vi "test_vision.vi"(11 "cam-id":T1="cam2") -> ()   [LabVIEW 2019]
uses:
  <vilib>/userDefined/High Color/IMAQdx.ctl
  Ctrl/clamp-result_cmd.ctl
  <vilib>/vision/driver/NI_Vision_Acquisition_Software.lvlib
  <resource>/objmgr/IMAQImage.rc
  <vilib>/vision/NI_Vision_Development_Module.lvlib
panel:
  in  "camera file":path
  in  "Reset":bool
  out "error out":errorcluster
  out "Steer Direction":dbl(slide)=22.0 scale=-30.0..30.0
  in  "weight_hor":dbl=0.5
  in  "camera_attrib":cluster{"brightness":u16, "exposure":dbl}={"brightness"=46, "exposure"=0.00510204081632653} {"exposure" scale=0.0..0.25; "brightness" scale=0.0..255.0}
  out "frame dt":u32=40
  out "loop n":i32=2970
  out "x-center":dbl=432.0
  out "dir-chart":cluster{dbl, "max angle":dbl}(graph)
  in  "Tab Control":T2(tab)
  out "dir-data":cluster{"Distance":sgl, "weight-dir":dbl}={"Distance"=506.17236, "weight-dir"=21.90533447265625} {"Distance" format="%.1f"; "weight-dir" format="%.1f"}
  in  "vertual speed":dbl(slide) scale=0.0..200.0
  out "Image roi-in":T3(plugin-control)
  out "Edge Coordinates":cluster{"X":sgl, "Y":sgl}[](array[cluster])=[{"X"=222.72447, "Y"=188.0}, {"X"=728.89685, "Y"=188.0}] {"Y" format="%.1f"; "X" format="%.1f"}
  in  "Clamp Settings":T4={"Contrast"=40, "Filter width"=4, "Steepness"=2, "Subsampling Ratio"=13, "Show Search Area"=TRUE, "Show Search Lines"=TRUE, "Show Edges Found"=TRUE, "Show Result"=TRUE}
  out "Image":T3(plugin-control)
  in  "Color Plane 2":i32(ring)=1 items=["Red", "Green", "Blue", "Hue", "Saturation", "Luminance", "Value", "Intensity"]
  out "ROI-clamp":T5={"Global Rectangle"=[62, 188, 838, 318], "Contours"=[{"Contour Type"=0, "ROI Type"=3, "Points"=[62, 188, 838, 318]}]}
  out "Image Size":cluster{"x":i32, "y":i32}={"x"=864, "y"=480}
  in  "stop":bool
  # "Camera ROI setting"
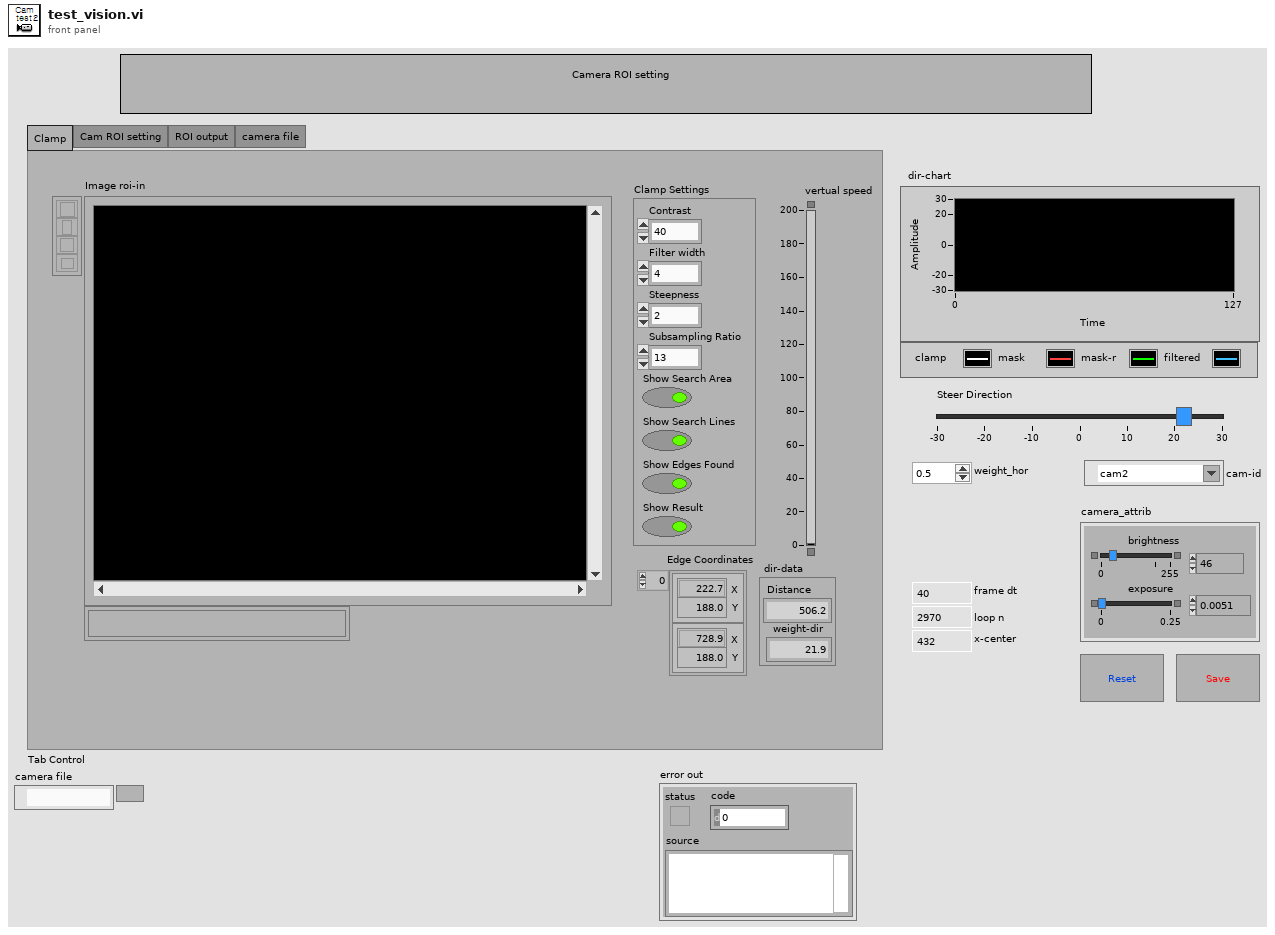
[diagram p1: front panel]
types:
  T1 = typedef "IMAQdx.ctl" = refnum<k21>
  T2 = enum32{"Clamp", "Cam ROI setting", "ROI output", "camera file"}
  T3 = typedef "IMAQ Image.ctl" = refnum<image>
  T4 = cluster{"Contrast":i32, "Filter width":i32, "Steepness":i32, "Subsampling Ratio":u32, "Show Search Area":bool, "Show Search Lines":bool, "Show Edges Found":bool, "Show Result":bool}
  T5 = cluster{"Global Rectangle":i32[], "Contours":cluster{"Contour Type":u32, "ROI Type":u32, "Points":i32[]}[]}
  T6 = typedef "clamp-result_cmd.ctl" = enum16{"write_clamp_overlay-result", "write_center-distance", "write_clamp_result", "write_threshold_result", "read"}
  T7 = typedef "IMAQ Rectangle" = cluster{"Left":i32, "Top":i32, "Right":i32, "Bottom":i32, "Rotation":dbl}
  T8 = typedef "ROI Descriptor" = cluster{"Global Rectangle":i32[], "Contours":cluster{"ID":enum32{"External", "Internal"}, "Type":u32, "Coordinates":i32[]}[]}
  T9 = cluster{"Points":cluster{"X":sgl, "Y":sgl}[], cluster{"X":sgl, "Y":sgl}[], cluster{cluster{"X":sgl, "Y":sgl}, cluster{"X":sgl, "Y":sgl}}[], "Perpendicular Lines":cluster{cluster{"X":sgl, "Y":sgl}, cluster{"X":sgl, "Y":sgl}}[], "ROI Descriptor out":T8}
  T10 = cluster{"Edge Coordinates":cluster{"X":sgl, "Y":sgl}[], "dir-data":cluster{"Distance":sgl, "weight-dir":dbl}, "clamp_result":cluster{"Points":cluster{"X":sgl, "Y":sgl}[], cluster{"X":sgl, "Y":sgl}[], cluster{cluster{"X":sgl, "Y":sgl}, cluster{"X":sgl, "Y":sgl}}[], "Perpendicular Lines":cluster{cluster{"X":sgl, "Y":sgl}, cluster{"X":sgl, "Y":sgl}}[], "ROI Descriptor out":T8}}
  T11 = cluster{"Edge Coordinates":cluster{"X":sgl, "Y":sgl}[], "dir-data":cluster{"Distance":sgl, "weight-dir":dbl}, "clamp_result":cluster{"Points-1":cluster{"X":sgl, "Y":sgl}[], "Points-2":cluster{"X":sgl, "Y":sgl}[], "Points-3":cluster{cluster{"X":sgl, "Y":sgl}, cluster{"X":sgl, "Y":sgl}}[], "Perpendicular Lines":cluster{cluster{"X":sgl, "Y":sgl}, cluster{"X":sgl, "Y":sgl}}[], "ROI Descriptor out":T8}}
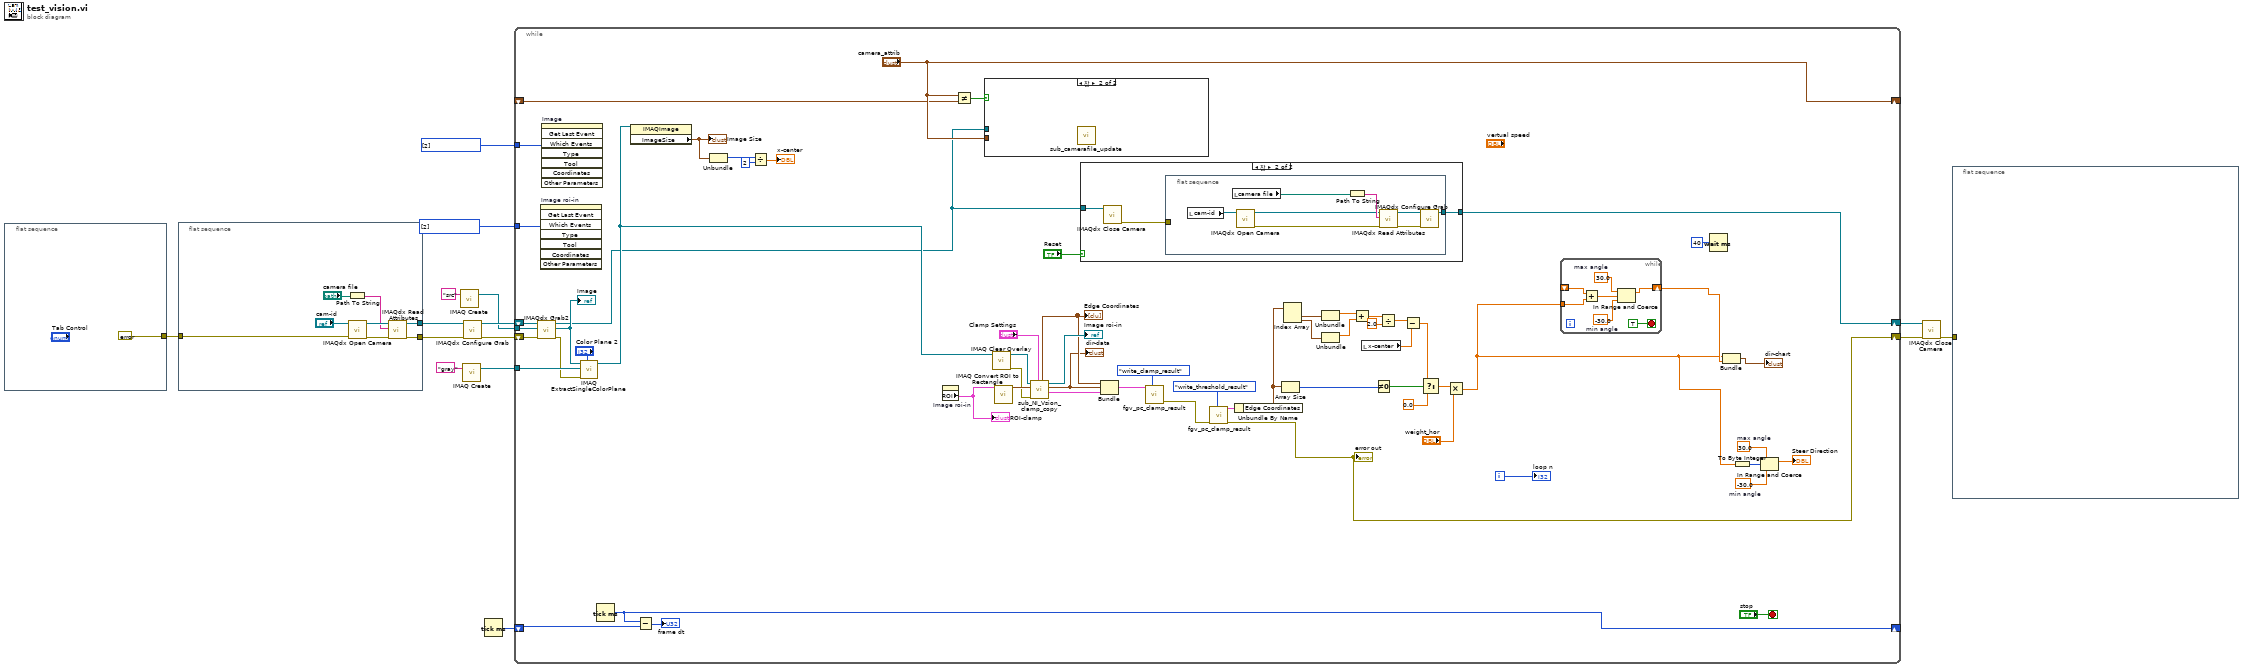
[diagram p0: block diagram]
diagram:
  w9 = i32[] [2] items=["No Event"=0, "Click Event"=1, "Draw Event"=2, "Size Event"=4, "Scroll Event"=5, "Double Click Event"=8] ("Which Events")
  w12 = i32[] [2] items=["No Event"=0, "Click Event"=1, "Draw Event"=2, "Size Event"=4, "Scroll Event"=5, "Double Click Event"=8] ("Which Events")
  n1 = flat-sequence {
    tunnel: [errorcluster {"status"=FALSE, "code"=0, "source"=""} ("error in")] -> w6
    frame #0 {
    }
  }
  n2 = flat-sequence {
    tunnel: [w22] -> w4
    tunnel: [w21] -> w10
    tunnel: w6 -> [w18]
    frame #0 {
      n3 = Path To String(path="camera file") -> (string=w20:string)
      n4 = call <vilib>:"IMAQdx Open Camera.vi"("error in"=w18, "Session In"="cam-id") -> ("error out"=w23:errorcluster, "Session Out"=w24:T1)  [unwired: 8 in]
      n5 = call <vilib>:"IMAQdx Read Attributes.vi"("error in"=w23, "Filename"=w20, "Session In"=w24) -> ("error out"=w21:errorcluster, "Session Out"=w22:T1)  [unwired: 7 in]
    }
  }
  n6 = call "IMAQ Create"("Image Name"="src") -> ("New Image"=w5:T3)  [unwired: 4 in, 1 out]
  n7 = call "IMAQ Create"("Image Name"="gray") -> ("New Image"=w13:T3)  [unwired: 4 in, 1 out]
  n8 = call <vilib>:"IMAQdx Configure Grab.vi"("error in"=w10, "Session In"=w4) -> ("error out"=w3:errorcluster, "Session Out"=w11:T1)  [unwired: 8 in]
  n9 = Tick Count (ms)() -> (millisecond timer value=w8:u32)
  n10 = while {
    tunnel: w5 -> [w83]
    tunnel: w13 -> [w64]
    tunnel: w12 -> [w87]
    tunnel: w9 -> [w81]
    shift-right: [w78] -> _
    shift-left: w8 -> [w79]
    shift-right: ["camera_attrib"] -> _
    shift-left: _ -> [w71]
    shift-right: [w31] -> w2
    shift-left: w11 -> [w82]
    shift-right: [w27] -> w1
    shift-left: w3 -> [w38]
    i -> [w84]
    stop <- "stop" stop-if-true
    w69 = -30.0  # min angle
    w68 = 30.0  # max angle
    n11 = call <vilib>:"IMAQdx Grab2.vi"("error in"=w38, "Image In"=w83, "Session In"=w82) -> ("error out"=w35:errorcluster, "Image Out"=w80:T3, "Session Out"=w32:T1)  [unwired: 5 in, 1 out]
    "Image" <- w80
    n12 = invoke on="Image roi-in" class="ImageControl" method="Get Last Event"("Which Events"=w81) -> ()  [unwired: 7 in, 8 out]
    n13 = invoke on="Image" class="ImageControl" method="Get Last Event"("Which Events"=w87) -> ()  [unwired: 7 in, 8 out]
    n14 = call "IMAQ ExtractSingleColorPlane"("Color Plane"="Color Plane 2", "error in (no error)"=w35, "Image Dst"=w64, "Image Src"=w80) -> ("Image Dst Out"=w36:T3)  [unwired: 6 in, 1 out]
    n15 = Tick Count (ms)() -> (millisecond timer value=w78:u32)
    n16 = property class="IMAQImage"(reference=w36) -> ("ImageSize"=w75:cluster{"x":i32, "y":i32})  [unwired: 1 in, 2 out]
    "Image Size" <- w75
    n17 = Subtract(x=w78, y=w79) -> (x-y=→"frame dt":u32)
    n18 = Unbundle(w75) -> ("x"=w76:i32)  [unwired: 1 out]
    n19 = Divide(x=w76, y=2) -> (x/y=→"x-center":dbl)
    n20 = property on="Image roi-in" class="ImageControl"() -> ("ROI"=w65:T5)  [unwired: 2 in, 2 out]
    "ROI-clamp" <- w65
    n21 = Not Equal?(x="camera_attrib", y=w71) -> (x != y?=w70:bool)
    n22 = case shown="참" w70 {
      tunnel: "camera_attrib" -> [_ _]
      tunnel: w32 -> [_ _]
      frame False {
      }
      frame True {
        n23 = call "sub_camerafile_update.vi"() -> ()  [unwired: 12 in]
      }
    }
    n24 = call "IMAQ Clear Overlay"("Image"=w36) -> ("error out"=w37:errorcluster, "Image Out"=w59:T3)  [unwired: 9 in]
    n25 = call "IMAQ Convert ROI to Rectangle"("ROI Descriptor"=w65) -> ("Rectangle"=w62:T7)  [unwired: 8 in, 1 out]
    n26 = call "sub_NI_Vsion_clamp_copy.vi"("Settings"="Clamp Settings", "error in (no error)"=w37, "Rectangle"=w62, "Image"=w59) -> ("clamp_result"=w58:T9, "dir-data"=w28:cluster{"Distance":sgl, "weight-dir":dbl}, "Image Out"=→"Image roi-in":T3, "Edge Coordinates"=w56:cluster{"X":sgl, "Y":sgl}[])  [unwired: 3 in, 1 out]
    "Edge Coordinates" <- w56
    "dir-data" <- w28
    n27 = case shown="참" "Reset" {
      tunnel: w32 -> [w88 w91]
      tunnel: [w88 w90] -> w31
      frame False {
      }
      frame True {
        n28 = call <vilib>:"IMAQdx Close Camera.vi"("Session In"=w91) -> ("error out"=w89:errorcluster)  [unwired: 10 in]
        n29 = flat-sequence {
          tunnel: [w95] -> w90
          tunnel: w89 -> [_]
          frame #0 {
            n30 = local read "cam-id"() -> (w99:T1)
            n31 = local read "camera file"() -> (w92:path)
            n32 = call <vilib>:"IMAQdx Open Camera.vi"("Session In"=w99) -> ("error out"=w94:errorcluster, "Session Out"=w93:T1)  [unwired: 9 in]
            n33 = Path To String(path=w92) -> (string=w98:string)
            n34 = call <vilib>:"IMAQdx Read Attributes.vi"("error in"=w94, "Filename"=w98, "Session In"=w93) -> ("error out"=w96:errorcluster, "Session Out"=w97:T1)  [unwired: 7 in]
            n35 = call <vilib>:"IMAQdx Configure Grab.vi"("error in"=w96, "Session In"=w97) -> ("Session Out"=w95:T1)  [unwired: 8 in, 1 out]
          }
        }
      }
    }
    n36 = Bundle("Edge Coordinates"=w56, "dir-data"=w28, "clamp_result"=w58) -> (w55:T10)  [unwired: 1 in]
    n37 = call "fgv_pc_clamp_result.vi"("cmd"=clamp-result_cmd."write_clamp_result", "clamp result in"=w55) -> ("error out"=w57:errorcluster)  [unwired: 6 in, 3 out]
    n38 = call "fgv_pc_clamp_result.vi"("cmd"=clamp-result_cmd."write_threshold_result", "error in"=w57) -> ("error out"=w27:errorcluster, "clamp result out"=w54:T11)  [unwired: 6 in, 2 out]
    "error out" <- w27
    n39 = Unbundle By Name(w54) -> ("Edge Coordinates"=w45:cluster{"X":sgl, "Y":sgl}[])
    n40 = Array Size(array=w45) -> (size(s)=w44:i32)
    n41 = Index Array(array=w45) -> (element #1=w53:cluster{"X":sgl, "Y":sgl}, element #2=w52:cluster{"X":sgl, "Y":sgl})  [unwired: 2 in]
    n42 = Unbundle(w53) -> ("X"=w51:sgl)  [unwired: 1 out]
    n43 = Unbundle(w52) -> ("X"=w50:sgl)  [unwired: 1 out]
    n44 = Add(x=w51, y=w50) -> (x+y=w49:sgl)
    n45 = local read "x-center"() -> (w46:dbl)
    n46 = Not Equal To 0?(x=w44) -> (x != 0?=w43:bool)
    n47 = Divide(x=w49, y=sgl 2.0) -> (x/y=w47:sgl)
    n48 = Subtract(x=w47, y=w46) -> (x-y=w41:dbl)
    n49 = Select(t=w41, s=w43, f=0.0 ("t")) -> (s? t:f=w40:dbl)
    n50 = Multiply(x=w40, y="weight_hor") -> (x*y=w26:dbl)
    n51 = while {
      shift-right: [w103] -> w34
      shift-left: _ -> [w105]
      tunnel: w26 -> [w106]
      stop <- TRUE stop-if-true
      w101 = -30.0  # min angle
      w102 = 30.0  # max angle
      n52 = Add(x=w105, y=w106) -> (x+y=w104:dbl)
      n53 = In Range and Coerce(upper limit=w102, x=w104, lower limit=w101) -> (coerced(x)=w103:dbl)  [unwired: 1 out]
    }
    n54 = Wait (ms)(milliseconds to wait=u32 40 ("delay")) -> ()  [unwired: 1 out]
    n55 = Bundle(w26, "max angle"=w34) -> (→"dir-chart":cluster{dbl, "max angle":dbl})  [unwired: 1 in]
    n56 = To Byte Integer(number=w26) -> (8bit integer=w66:i8)
    n57 = In Range and Coerce(upper limit=w68, x=w66, lower limit=w69) -> (coerced(x)=→"Steer Direction":dbl)  [unwired: 1 out]
    "loop n" <- w84
  }
  n58 = call <vilib>:"IMAQdx Close Camera.vi"("error in"=w1, "Session In"=w2) -> ("error out"=w7:errorcluster)  [unwired: 9 in]
  n59 = flat-sequence {
    tunnel: w7 -> [_]
    frame #0 {
    }
  }
